vi "BGInfo.vi"() -> ()   [LabVIEW 2019]
uses:
  <userlib>/APTLib.lnk/File IO/_Read Write Data File _APTLib.llb/File IO Option _APTLib.ctl
  <userlib>/APTLib.lnk/File IO/_Read Write Data File _APTLib.llb/Text Encoding Format _APTLib.ctl
  <userlib>/APTLib.lnk/File IO/_Read Write Data File _APTLib.llb/Read Write Unicode Text File _APTLib.vi
  <userlib>/APTLib.lnk/File IO/Path Operations/_Extension _APTLib.llb/Append Extension(string) _APTLib.vi
panel:
  in  "#Kural":i32=1330
  out "error out":errorcluster
  out "Data":string
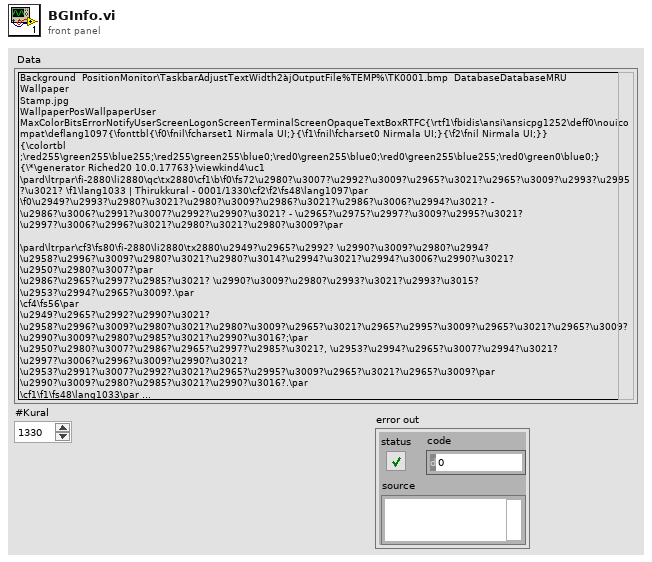
[diagram p1: front panel]
types:
  T1 = typedef "Text Encoding Format _APTLib.ctl" = enum8{"ASCII", "UTF-8", "UTF-16 LE", "UTF-16 BE"}
  T2 = typedef "File IO Option _APTLib.ctl" = enum16{"Read", "Write"}
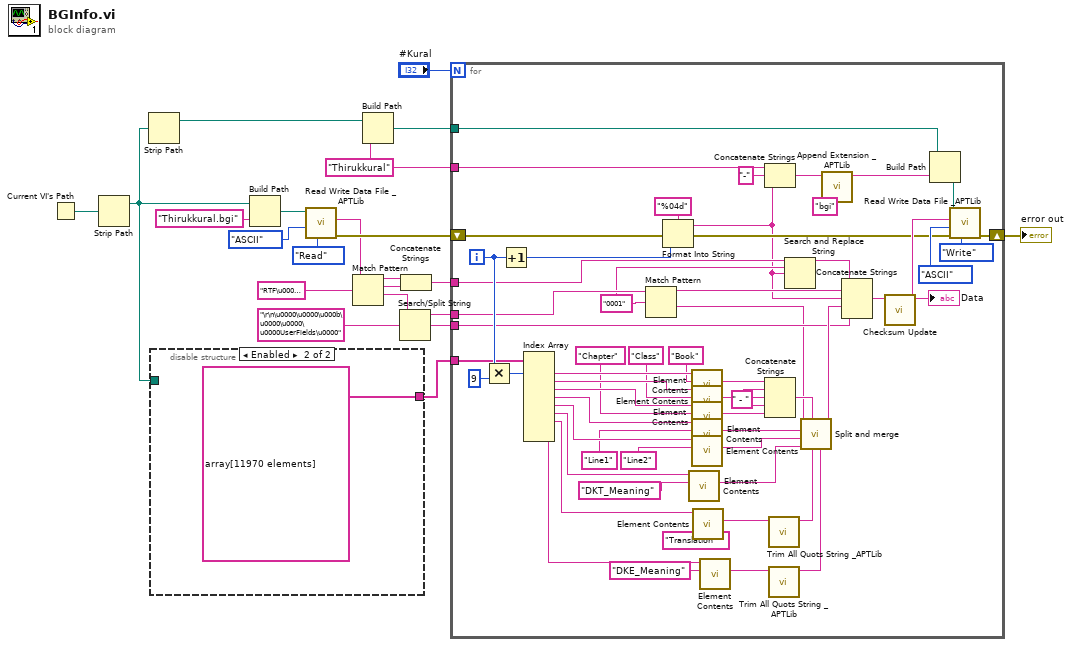
[diagram p0: block diagram]
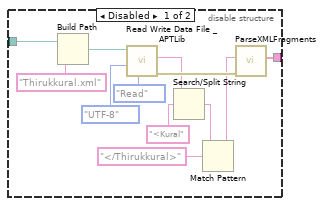
[diagram p2: hidden frame]
diagram:
  w2 = "Thirukkural" ("name or relative path")
  n1 = Current VI's Path() -> (path=w8:path)
  n2 = Strip Path(path=w8) -> (stripped path=w3:path)  [unwired: 1 out]
  n3 = Strip Path(path=w3) -> (stripped path=w7:path)  [unwired: 1 out]
  n4 = disable-structure shown="Enabled" {
    disable-tunnel: [w33 string[] array[11970 elements] ("XML Elements")] -> w10
    disable-tunnel: w3 -> [w24 _]
    frame Disabled {
      n5 = Build Path(base path=w24, name or relative path="Thirukkural.xml") -> (appended path=w23:path)
      n6 = call-poly <userlib>:"Read Write Data File _APTLib.vi"("Option"=File_IO_Option__APTLib."Read", "Encoding?"=Text_Encoding_Format__APTLib."UTF-8", "file path"=w23) -> ("error out"=w30:errorcluster, "String Out"=w28:string)  [unwired: 6 in, 1 out]
      n7 = Search/Split String(string=w28, search string/char (-)="<Kural") -> (match + rest of string=w26:string)  [unwired: 1 in, 2 out]
      n8 = Match Pattern(string=w26, regular expression="</Thirukkural>" ("Substring")) -> (before substring=w29:string)  [unwired: 1 in, 3 out]
      n9 = call <vilib>:"ParseXMLFragments.vi"("error in (no error)"=w30, "XML in"=w29) -> ("XML Elements"=w33:string[])  [unwired: 8 in, 1 out]
    }
    frame Enabled {
    }
  }
  n10 = Build Path(base path=w3, name or relative path="Thirukkural.bgi" ("File Name")) -> (appended path=w20:path)
  n11 = call-poly <userlib>:"Read Write Data File _APTLib.vi"("Option"=File_IO_Option__APTLib."Read", "Encoding?"=Text_Encoding_Format__APTLib."ASCII", "file path"=w20) -> ("error out"=w19:errorcluster, "String Out"=w16:string)  [unwired: 6 in, 1 out]
  n12 = Match Pattern(string=w16, regular expression="RTF\u0000\u0001\u0000\u0000\u0000" ("search string/char (-)")) -> (before substring=w15:string, match substring=w13:string, after substring=w12:string)  [unwired: 1 in, 1 out]
  n13 = Build Path(base path=w7, name or relative path=w2) -> (appended path=w5:path)
  n14 = Search/Split String(string=w12, search string/char (-)="\r\n\u0000\u0000\u000b\u0000\u0000\u0000UserFields\u0000") -> (substring before match=w11:string, match + rest of string=w6:string)  [unwired: 1 in, 1 out]
  n15 = Concatenate Strings(w15, w13) -> (w14:string)
  n16 = for {
    N: "#Kural" -> [_]
    tunnel: w2 -> [w55]
    tunnel: w14 -> [w48]
    tunnel: w11 -> [w51]
    tunnel: w6 -> [w60]
    tunnel: w10 -> [w84]
    shift-right: [w83] -> w9
    shift-left: w19 -> [w53]
    tunnel: w5 -> [w80]
    i -> [w86]
    w47 = "0001" ("regular expression")
    w57 = " - " ("string")
    n17 = Multiply(x=w86, y=9) -> (x*y=w72:i32)
    n18 = Increment(x=w86) -> (x+1=w88:i32)
    n19 = Index Array(array=w84, index #1=w72) -> (element #1=w71:string, element #2=w70:string, element #3=w69:string, element #4=w77:string, element #5=w79:string, element #6=w39:string, element #7=w40:string, element #9=w37:string)  [unwired: 8 in, 1 out]
    n20 = Match Pattern(string=w51, regular expression=w47) -> (before substring=w49:string, after substring=w50:string)  [unwired: 1 in, 2 out]
    n21 = Format Into String(format string="%04d", error in=w53, w88) -> (resulting string=w45:string, error out=w61:errorcluster)  [unwired: 1 in]
    n22 = call "Element Contents.vi"("Name"="DKT_Meaning" ("Substring"), "XML in"=w39) -> ("Content"=w36:string)  [unwired: 8 in, 1 out]
    n23 = call "Element Contents.vi"("Name"="Book", "XML in"=w71) -> ("Content"=w65:string)  [unwired: 8 in, 1 out]
    n24 = call "Element Contents.vi"("Name"="Class", "XML in"=w70) -> ("Content"=w64:string)  [unwired: 8 in, 1 out]
    n25 = call "Element Contents.vi"("Name"="Chapter", "XML in"=w69) -> ("Content"=w63:string)  [unwired: 8 in, 1 out]
    n26 = call "Element Contents.vi"("Name"="Line1", "XML in"=w77) -> ("Content"=w75:string)  [unwired: 8 in, 1 out]
    n27 = call "Element Contents.vi"("Name"="Line2" ("Substring"), "XML in"=w79) -> ("Content"=w74:string)  [unwired: 8 in, 1 out]
    n28 = call "Element Contents.vi"("Name"="Translation", "XML in"=w40) -> ("Content"=w42:string)  [unwired: 8 in, 1 out]
    n29 = call "Element Contents.vi"("Name"="DKE_Meaning", "XML in"=w37) -> ("Content"=w44:string)  [unwired: 8 in, 1 out]
    n30 = Concatenate Strings(w55, "-" ("string"), w45) -> (w54:string)
    n31 = Concatenate Strings(w65, w57, w64, w57, w63) -> (w58:string)
    n32 = call "Trim All Quots String _APTLib.vi"("String In"=w42) -> ("String Out"=w41:string)  [unwired: 10 in]
    n33 = call "Trim All Quots String _APTLib.vi"("String In"=w44) -> ("String Out"=w43:string)  [unwired: 10 in]
    n34 = Search and Replace String(input string=w48, search string=w47, replace string=w45) -> (result string=w46:string)  [unwired: 5 in, 3 out]
    n35 = call "Split and merge.vi"("DKE_Meaning"=w43, "Translation"=w41, "Index"=w58, "DKT_Meaning"=w36, "Line 2"=w74, "Line1"=w75, "String In"=w50) -> ("String Output"=w81:string)  [unwired: 4 in]
    n36 = call-poly <userlib>:"Append Extension _APTLib.vi"("Extension"="bgi" ("File Name"), "File Name"=w54) -> ("File Name with Extension"=w91:string)  [unwired: 9 in]
    n37 = Concatenate Strings(w46, w49, w45, w81, w60) -> (w73:string)
    n38 = call "Checksum Update.vi"("BGI Data In"=w73) -> ("BGI Data Out"=w62:string)  [unwired: 9 in, 1 out]
    "Data" <- w62
    n39 = Build Path(base path=w80, name or relative path=w91) -> (appended path=w90:path)
    n40 = call-poly <userlib>:"Read Write Data File _APTLib.vi"("Option"=File_IO_Option__APTLib."Write", "error in"=w61, "Encoding?"=Text_Encoding_Format__APTLib."ASCII", "String In"=w62, "file path"=w90) -> ("error out"=w83:errorcluster)  [unwired: 4 in, 2 out]
  }
  "error out" <- w9
